vi "Assert Collection Distinct.vi"(7 "Message (\"\")":string, 8 "error in (no error)":errorcluster, 10 "Collection":variant) -> (0 "error out":errorcluster)   [LabVIEW 2017, in "Transparent Assertions.lvlib"]
doc: "Asserts that all elements in a collection (array or map) are distinct. Returns an error if the assertion fails, and optionally appends a custom message to the error.\n\nFor maps, the values are compared for distinctness.\n\nThis assertion is not needed for sets, because sets can only contain distinct elements by definition."
uses:
  Transparent Assertions.lvlib
  Collection Distinct/Collection Distinct.lvclass
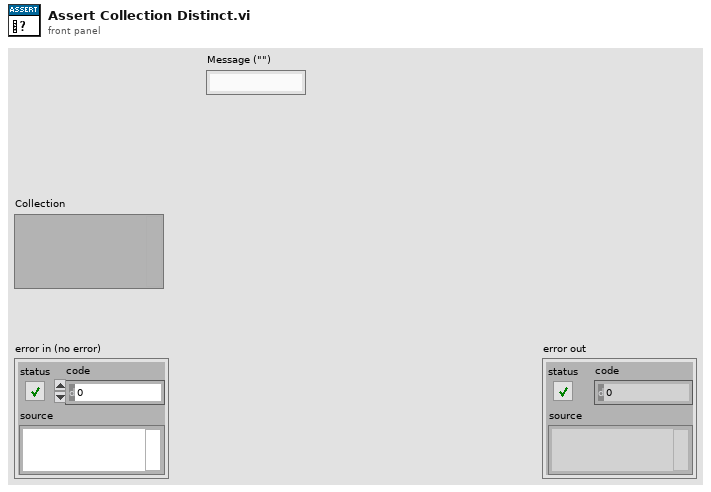
[diagram p1: front panel]
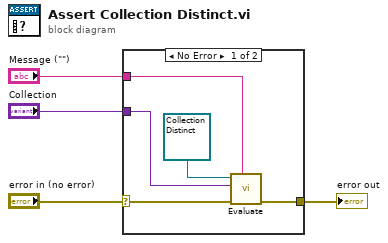
[diagram p0: block diagram]
diagram:
  n1 = case shown="No Error" "error in (no error)" {
    selector: "error in (no error)" -> [w6 w10]
    tunnel: [w9 w10] -> w4
    tunnel: "Collection" -> [w8 _]
    tunnel: "Message (\"\")" -> [w7 _]
    frame No Error {
      n2 = call-dynamic "Evaluate.vi"("Message (\"\")"=w7, "error in (no error)"=w6, "Actual"=w8, "Constraint in"=refnum<class "Collection Distinct.lvclass"> refnum ("Transparent Assertions.lvlib:Constraints.lvlib:Collection Distinct.lvclass")) -> ("error out"=w9:errorcluster)  [unwired: 6 in, 1 out]
    }
    frame Error {
    }
  }
  "error out" <- w4
